vi "LoRa Air-Time Calculator.vi"() -> ()   [LabVIEW 2021]
panel:
  out "Throughput (bps)":dbl format="%#.3f"
  out "Payload Time Time (ms)":dbl format="%#.3f"
  out "Preamble Time (ms)":dbl format="%#.3f"
  out "Preamble Number":dbl format="%#.3f"
  out "Symbol Rate":dbl format="%#.3f"
  out "Air-Time (ms)":dbl format="%#.3f"
  out "Payload (Symbol)":dbl
  out "Symbol Time (ms)":dbl format="%#.3g"
  in  "Low Data Rate Optimization":bool
  in  "Explicit Header":bool
  in  "CRC":bool
  in  "Coding Rate":u32(ring)=5 items=["4/5"=5, "4/6"=6, "4/7"=7, "4/8"=8]
  in  "Bandwidth":u32(ring)=500000 items=["7.8 KHz"=7800, "10.4 KHz"=10400, "15.6 KHz"=15600, "20.8 KHz"=20800, "31.2 KHz"=31200, "41.7 KHz"=41700, "62.5 KHz"=62500, "125 KHz"=125000, "250 KHz"=250000, "500 KHz"=500000]
  in  "Spreading Factor":u16(ring)=6 items=["6"=6, "7"=7, "8"=8, "9"=9, "10"=10, "11"=11, "12"=12]
  in  "Preamble Size":u16=6 min=6 step=1
  in  "Payload Size":u8=1 min=1 step=1
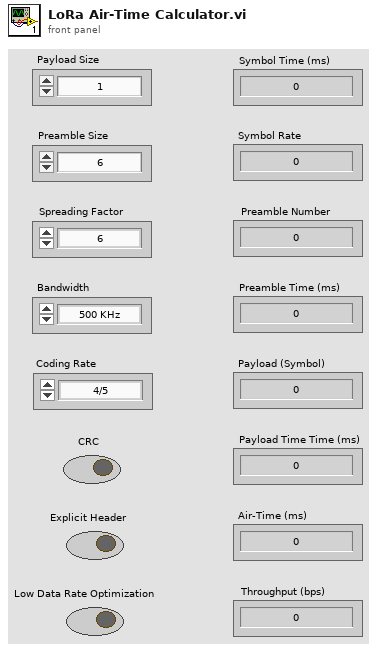
[diagram p1: front panel]
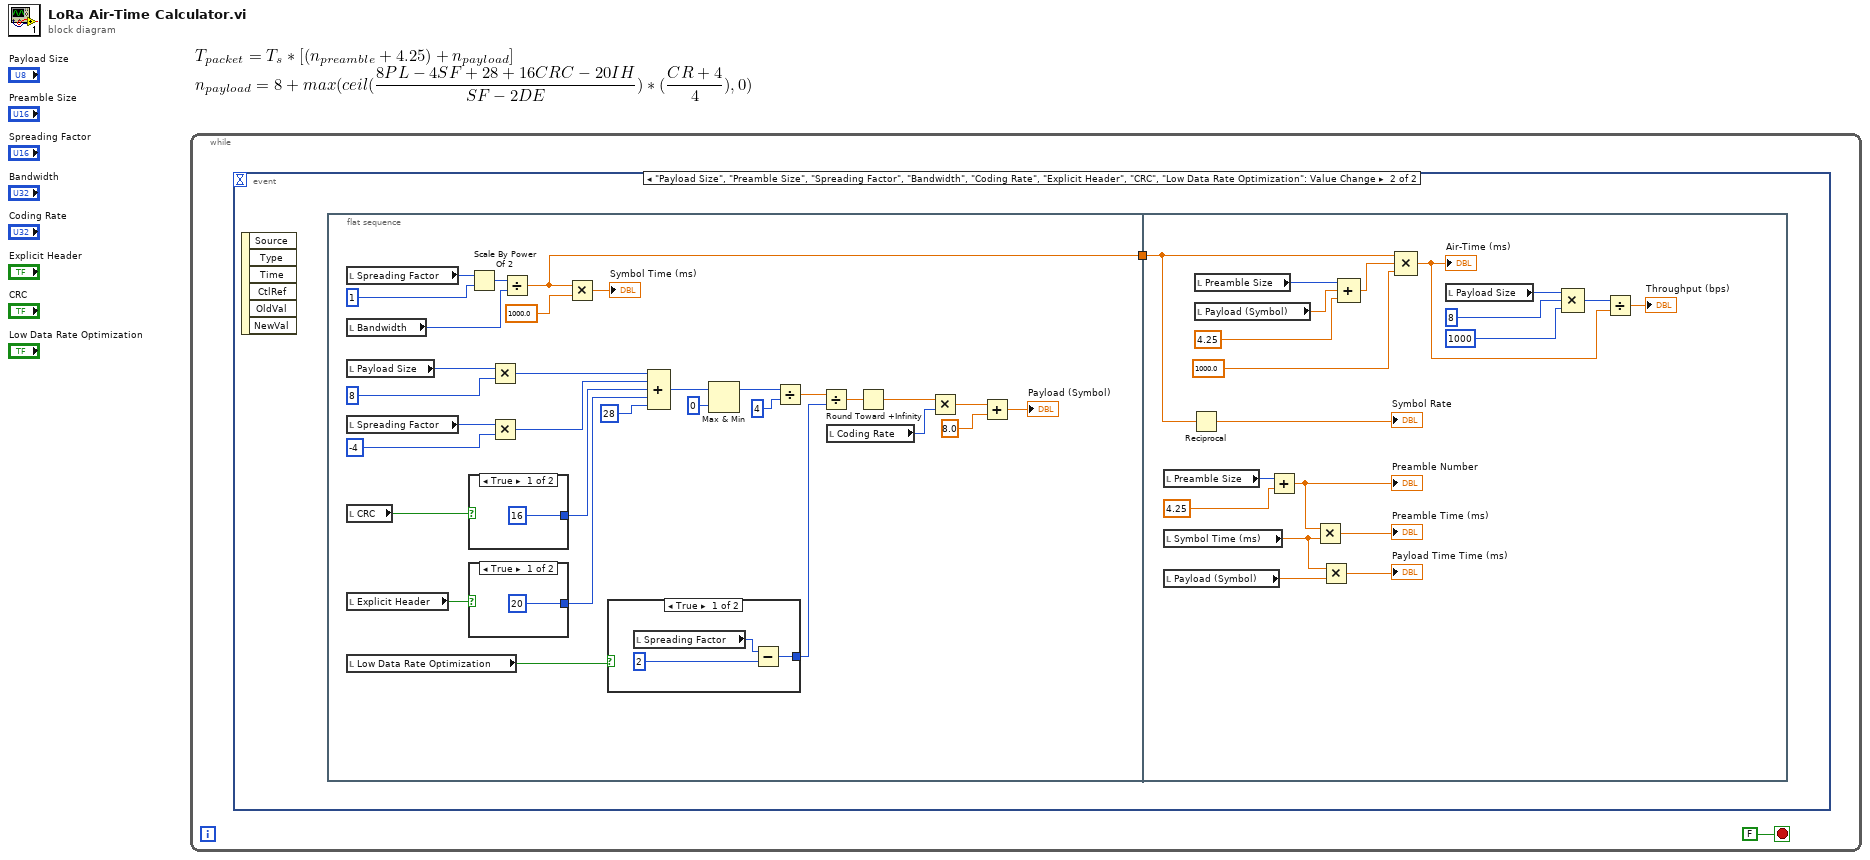
[diagram p0: block diagram]
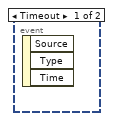
[diagram p2: hidden frame]
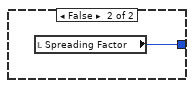
[diagram p3: hidden frame]
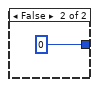
[diagram p4: hidden frame]
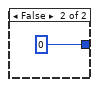
[diagram p5: hidden frame]
diagram:
  n1 = while {
    stop <- FALSE stop-if-true
    n2 = event shown="[1] \"Payload Size\", \"Preamble Size\", \"Spreading Factor\", \"Bandwidth\", \"Coding Rate\", \"Explicit Header\", \"CRC\", \"Low Data Rate Optimization\": Value Change" {
      selector: _ -> [_ _]
      dyn-events: _ -> [_ _]
      timeout: _ -> [_ _]
      event Timeout {
        n3 = event-data() -> ()  [unwired: 1 in, 3 out]
      }
      event "Payload Size", "Preamble Size", "Spreading Factor", "Bandwidth", "Coding Rate", "Explicit Header", "CRC", "Low Data Rate Optimization": Value Change {
        n4 = event-data() -> ()  [unwired: 1 in, 6 out]
        n5 = flat-sequence {
          tunnel: [w3] -> w2
          tunnel: w2 -> [w56]
          frame #0 {
            n6 = local read "Spreading Factor"() -> (w7:u16)
            n7 = local read "Bandwidth"() -> (w9:u32)
            n8 = local read "Payload Size"() -> (w33:u8)
            n9 = local read "Spreading Factor"() -> (w31:u16)
            n10 = local read "CRC"() -> (w29:bool)
            n11 = local read "Explicit Header"() -> (w28:bool)
            n12 = local read "Low Data Rate Optimization"() -> (w20:bool)
            n13 = Scale By Power Of 2(n=w7, x=1) -> (x*2^n=w8:i32)
            n14 = case shown="True" w29 {
              tunnel: [16 ("y") 0 ("y")] -> w25
              frame True {
              }
              frame False {
              }
            }
            n15 = case shown="True" w28 {
              tunnel: [20 ("y") 0 ("y")] -> w24
              frame True {
              }
              frame False {
              }
            }
            n16 = Multiply(x=w33, y=8) -> (x*y=w27:i32)
            n17 = Multiply(x=w31, y=-4) -> (x*y=w26:i32)
            n18 = Divide(x=w8, y=w9) -> (x/y=w3:dbl)
            n19 = Multiply(x=w3, y=1000.0) -> (x*y=→"Symbol Time (ms)":dbl)
            n20 = case shown="True" w20 {
              tunnel: [w34 w37] -> w16
              frame True {
                n21 = local read "Spreading Factor"() -> (w36:u16)
                n22 = Subtract(x=w36, y=u16 2) -> (x-y=w34:u16)
              }
              frame False {
                n23 = local read "Spreading Factor"() -> (w37:u16)
              }
            }
            n24 = Compound Arithmetic op=ADD(w27, w26, w25, w24, 28 ("value")) -> (w22:i32)
            n25 = Max & Min(x=w22, y=0) -> (max(x,y)=w19:i32)  [unwired: 1 out]
            n26 = Divide(x=w19, y=4) -> (x/y=w17:dbl)
            n27 = Divide(x=w17, y=w16) -> (x/y=w15:dbl)
            n28 = local read "Coding Rate"() -> (w13:u32)
            n29 = Round Toward +Infinity(x=w15) -> (ceil(x): smallest int >= x=w14:dbl)
            n30 = Multiply(x=w14, y=w13) -> (x*y=w12:dbl)
            n31 = Add(x=w12, y=8.0) -> (x+y=→"Payload (Symbol)":dbl)
          }
          frame #1 {
            n32 = local read "Preamble Size"() -> (w54:u16)
            n33 = local read "Symbol Time (ms)"() -> (w50:dbl)
            n34 = local read "Payload (Symbol)"() -> (w49:dbl)
            n35 = Reciprocal(x=w56) -> (1/x=→"Symbol Rate":dbl)
            n36 = local read "Preamble Size"() -> (w61:u16)
            n37 = local read "Payload (Symbol)"() -> (w59:dbl)
            n38 = Add(x=w54, y=4.25) -> (x+y=w52:dbl)
            "Preamble Number" <- w52
            n39 = Multiply(x=w52, y=w50) -> (x*y=→"Preamble Time (ms)":dbl)
            n40 = Multiply(x=w50, y=w49) -> (x*y=→"Payload Time Time (ms)":dbl)
            n41 = Compound Arithmetic op=ADD(w61, w59, 4.25 ("y")) -> (w58:dbl)
            n42 = Compound Arithmetic op=MULTIPLY(w56, w58, 1000.0 ("y")) -> (w44:dbl)
            "Air-Time (ms)" <- w44
            n43 = local read "Payload Size"() -> (w47:u8)
            n44 = Compound Arithmetic op=MULTIPLY(w47, u8 8 ("y"), 1000 ("value")) -> (w45:i32)
            n45 = Divide(x=w45, y=w44) -> (x/y=→"Throughput (bps)":dbl)
          }
        }
      }
    }
  }
